vi "read dvr.vi"(6 "wait for reply (T)":bool=TRUE, 8 "error in":errorcluster, 11 "Module ID":i32=-1) -> (0 "error out":errorcluster, 1 "timed out?":bool, 2 "Numeric":dbl)   [LabVIEW 2025, in "Wheatstone Bridge.lvlib"]
doc: "_____\nCreated using DQMH Framework: Event Scripter 7.1.2.1547."
uses:
  Wheatstone Bridge.lvlib
  read dvr Argument--cluster.ctl
  read dvr (Reply Payload)--cluster.ctl
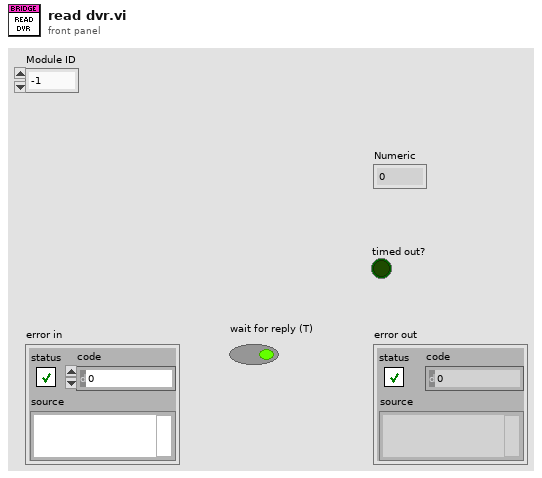
[diagram p1: front panel]
types:
  T1 = typedef "Wheatstone Bridge.lvlib/read dvr Argument--cluster.ctl" = cluster{"Module ID":i32, "Wait Notifier":refnum<notifier>, "wait for reply":bool}
  T2 = typedef "Wheatstone Bridge.lvlib/Request Events--cluster.ctl" = cluster{"Stop Module":refnum<user-event>, "Show Panel":refnum<user-event>, "Hide Panel":refnum<user-event>, "Show Diagram":refnum<user-event>, "Get Module Execution Status":refnum<user-event>, "select child":refnum<user-event>, "read config":refnum<user-event>, "init":refnum<user-event>, "init device":refnum<user-event>, "close":refnum<user-event>, "read data":refnum<user-event>, "read dvr":refnum<user-event>}
  T3 = typedef "Wheatstone Bridge.lvlib/read dvr (Reply Payload)--cluster.ctl" = cluster{"Module ID":i32, "Numeric":dbl, "error":errorcluster}
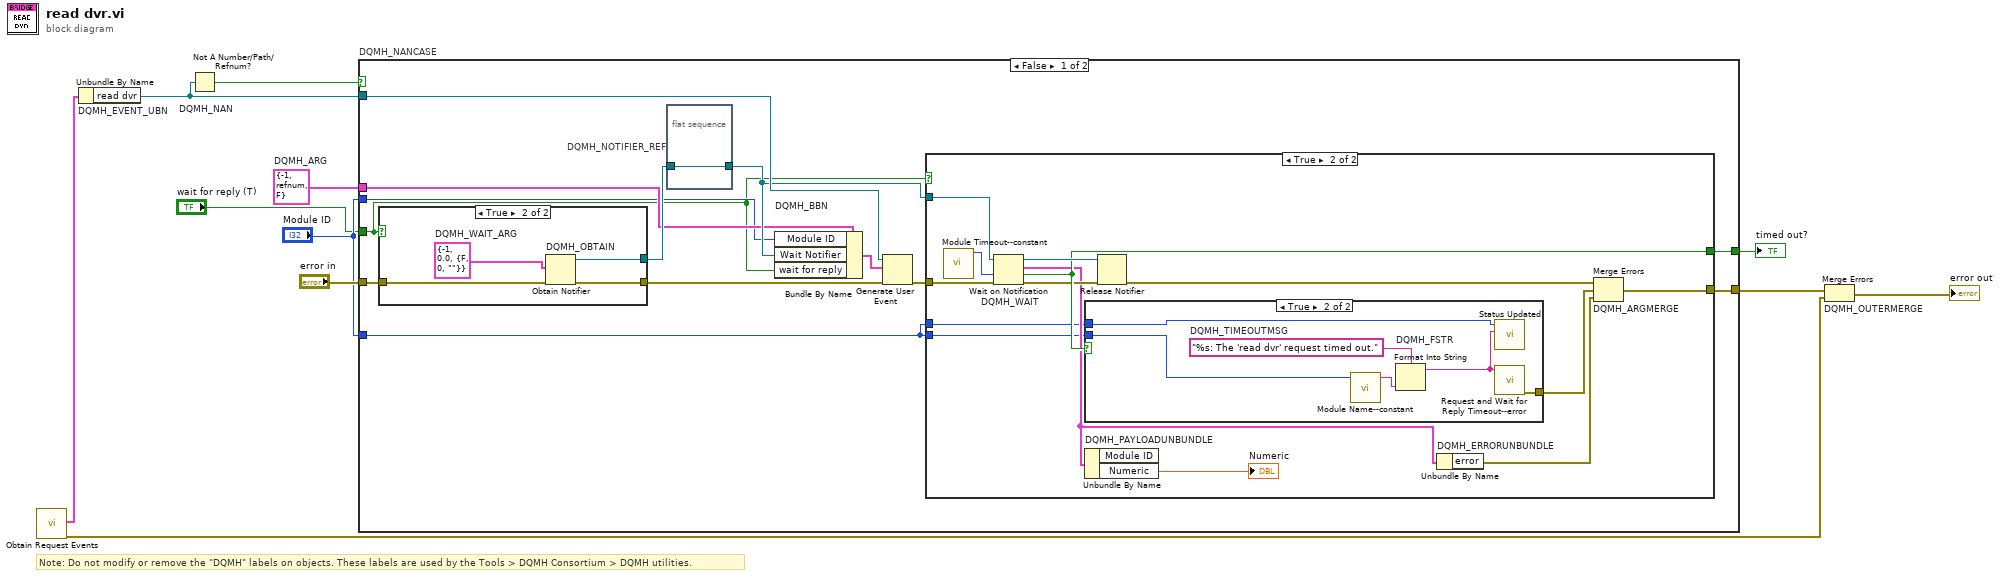
[diagram p0: block diagram]
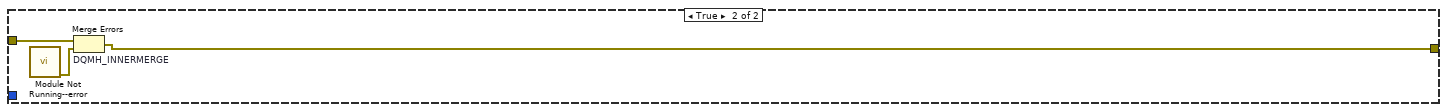
[diagram p5: hidden frame]
diagram:
  w5 = T1 {"Module ID"=-1, "Wait Notifier"=refnum, "wait for reply"=FALSE}  # DQMH_ARG
  # "Note: Do not modify or remove the \"DQMH\" labels on objects. These labels are used by the Tools > DQMH Consortium > DQMH utilities."
  n1 = call "Obtain Request Events.vi"() -> ("error out"=w2:errorcluster, "Wheatstone Bridge Request Events"=w1:T2)  [unwired: 10 in]
  n2 = Unbundle By Name "DQMH_EVENT_UBN"(w1) -> ("read dvr"=w9:refnum<user-event>)
  n3 = Not A Number/Path/Refnum? "DQMH_NAN"(number/path/refnum=w9) -> (NaN/Path/Refnum?=w8:bool)
  n4 = case "DQMH_NANCASE" shown="False" w8 {
    tunnel: "error in" -> [w24 w54]
    tunnel: w9 -> [w22 _]
    tunnel: [w19 w53] -> w6
    tunnel: [w20 _] -> w7
    tunnel: w5 -> [w15 _]
    tunnel: "Module ID" -> [w14 _]
    tunnel: "Module ID" -> [w13 _]
    tunnel: "wait for reply (T)" -> [w12 _]
    frame False {
      n5 = case shown="True" w12 {
        tunnel: w24 -> [w47 w51]
        tunnel: [w47 w50] -> w21
        tunnel: [_ w48] -> w17
        frame False {
        }
        frame True {
          w49 = T3 {"Module ID"=-1, "Numeric"=0.0, "error"={"status"=FALSE, "code"=0, "source"=""}}  # DQMH_WAIT_ARG
          n6 = Obtain Notifier "DQMH_OBTAIN"(notification data type=w49, error in (no error)=w51) -> (notifier out=w48:refnum<notifier>, error out=w50:errorcluster)  [unwired: 2 in, 1 out]
        }
      }
      n7 = flat-sequence "DQMH_NOTIFIER_REF" {
        tunnel: w17 -> [w25]
        tunnel: [w25] -> w16
        frame #0 {
        }
      }
      n8 = Bundle By Name "DQMH_BBN"(cluster=w15, "Module ID"=w14, "Wait Notifier"=w16, "wait for reply"=w12) -> (w18:T1)
      n9 = Generate User Event(user event=w22, event data cluster=w18, error in=w21) -> (error out=w23:errorcluster)  [unwired: 1 in, 1 out]
      n10 = case shown="True" w12 {
        tunnel: w23 -> [w26 w40]
        tunnel: w16 -> [_ w39]
        tunnel: [_ w37] -> w20
        tunnel: [w26 w36] -> w19
        tunnel: w13 -> [_ w28]
        tunnel: w13 -> [_ w27]
        frame False {
        }
        frame True {
          n11 = call "Module Timeout--constant.vi"() -> ("Module Timeout"=w30:i32)  [unwired: 11 in]
          n12 = Wait on Notification "DQMH_WAIT"(notifier=w39, timeout in ms (-1)=w30, error in (no error)=w40) -> (notifier out=w38:refnum<notifier>, notification=w31:T3, timed out?=w37:bool, error out=w35:errorcluster)  [unwired: 1 in]
          n13 = case shown="True" w37 {
            tunnel: [_ w44] -> w32
            tunnel: w28 -> [_ w42]
            tunnel: w27 -> [_ w41]
            frame False {
            }
            frame True {
              w46 = "%s: The 'read dvr' request timed out."  # DQMH_TIMEOUTMSG
              n14 = call "Module Name--constant.vi"("Module ID"=w41) -> ("Module Name"=w43:string)  [unwired: 10 in]
              n15 = Format Into String "DQMH_FSTR"(format string=w46, w43) -> (resulting string=w45:string)  [unwired: 2 in, 1 out]
              n16 = call "Status Updated.vi"("Status"=w45, "Module ID"=w42) -> ()  [unwired: 9 in, 1 out]
              n17 = call "Request and Wait for Reply Timeout--error.vi"("Error Message"=w45) -> ("error out"=w44:errorcluster)  [unwired: 10 in]
            }
          }
          n18 = Unbundle By Name "DQMH_PAYLOADUNBUNDLE"(w31) -> ("Numeric"=→"Numeric":dbl)  [unwired: 1 out]
          n19 = Release Notifier(notifier=w38, error in (no error)=w35) -> (error out=w34:errorcluster)  [unwired: 1 in, 2 out]
          n20 = Unbundle By Name "DQMH_ERRORUNBUNDLE"(w31) -> ("error"=w33:errorcluster)
          n21 = Merge Errors "DQMH_ARGMERGE"(w34, w32, w33) -> (w36:errorcluster)
        }
      }
    }
    frame True {
      n22 = call "Module Not Running--error.vi"() -> ("error out"=w52:errorcluster)  [unwired: 11 in]
      n23 = Merge Errors "DQMH_INNERMERGE"(w54, w52) -> (w53:errorcluster)
    }
  }
  "timed out?" <- w7
  n24 = Merge Errors "DQMH_OUTERMERGE"(w6, w2) -> (→"error out":errorcluster)
